vi "onStart.vi"(8 "error in (no error)":errorcluster, 11 "Instrument.Lockin":refnum<class "Instrument.Lockin.lvclass">) -> (0 "error out":errorcluster, 3 "Instrument.Lockin out":refnum<class "Instrument.Lockin.lvclass">)   [LabVIEW 2019, in "Instrument.Lockin.lvlib" / "Instrument.Lockin.lvclass"]
doc: "JKI State Machine Objects (SMO) 2.0.0.73\nJKI - JKI\nCopyright (c) 2025, JKI"
uses:
  Instrument.Lockin.lvclass
  <userlib>/LevyLab/Instrument Framework/Instrument Types/Lockin/Instrument.LockinAPI.lvclass
panel:
  # "For instructions on how to use the JKI State Machine Objects, examples and video tutorials, visit:\nhttp://jki.net/state-machine-objects/\n\nJKI State Machine Objects™\nhttp://jki.net/state-machine-objects/\nCopyright (C) 2005-2015, JKI <info@jki.net>\nALL RIGHTS RESERVED"
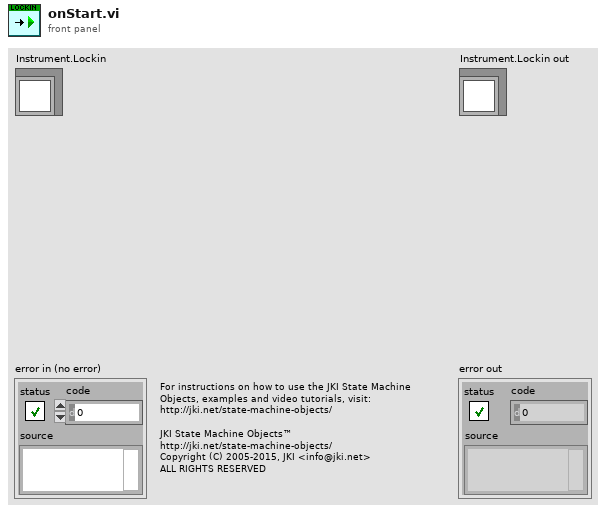
[diagram p1: front panel]
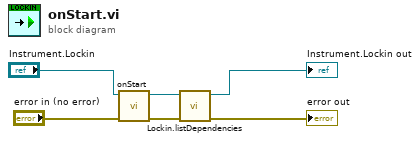
[diagram p0: block diagram]
diagram:
  n1 = call-parent "onStart.vi"("error in (no error)"="error in (no error)", "SMO"="Instrument.Lockin") -> ("error out"=w3:errorcluster, "SMO out"=w4:refnum<class "Instrument.Lockin.lvclass">)  [unwired: 8 in]
  n2 = call "Lockin.listDependencies.vi"("error in (no error)"=w3, "Instrument.Lockin in"=w4) -> ("error out"=→"error out":errorcluster, "Instrument.Lockin out"=→"Instrument.Lockin out":refnum<class "Instrument.Lockin.lvclass">)  [unwired: 7 in, 1 out]
